vi "TemperatureSetup (SubVI).vi"() -> (0 "error out":errorcluster, 3 "Refnum out":refnum<k21>)   [LabVIEW 2016]
uses:
  <vilib>/DAQmx/create/channels.llb/DAQmx Create Channel (AI-Temperature-Thermocouple).vi
  <resource>/objmgr/daqmx.rc
  <vilib>/DAQmx/configure/timing.llb/DAQmx Timing (Sample Clock).vi
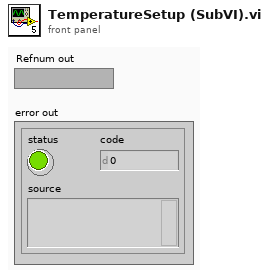
[diagram p1: front panel]
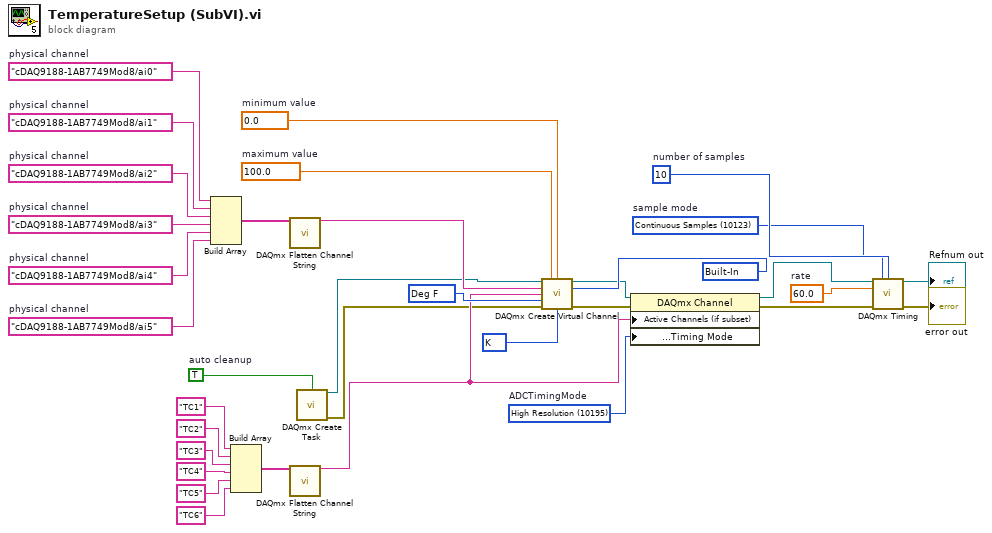
[diagram p0: block diagram]
diagram:
  w29 = "cDAQ9188-1AB7749Mod8/ai5"  # physical channel
  w28 = "cDAQ9188-1AB7749Mod8/ai4"  # physical channel
  w27 = "cDAQ9188-1AB7749Mod8/ai3"  # physical channel
  w26 = "cDAQ9188-1AB7749Mod8/ai2"  # physical channel
  w22 = "cDAQ9188-1AB7749Mod8/ai1"  # physical channel
  w21 = "cDAQ9188-1AB7749Mod8/ai0"  # physical channel
  w20 = 10144 items=["Deg C"=10143, "Deg F"=10144, "Kelvins"=10325, "Deg R"=10145, "From Custom Scale"=10065] ("units")
  w19 = 10073 items=["J"=10072, "K"=10073, "N"=10077, "R"=10082, "S"=10085, "T"=10086, "B"=10047, "E"=10055] ("thermocouple type")
  w18 = 10200 items=["Built-In"=10200, "Constant Value"=10116, "Channel"=10113] ("cjc source")
  w1 = 10123 items=["Finite Samples"=10178, "Continuous Samples"=10123, "Hardware Timed Single Point"=12522]  # sample mode
  w2 = 10  # number of samples
  w3 = 60.0  # rate
  w6 = 10195 items=["High Resolution"=10195, "High Speed"=14712, "Best 50 Hz Rejection"=14713, "Best 60 Hz Rejection"=14714]  # ADCTimingMode
  w9 = 0.0  # minimum value
  w10 = 100.0  # maximum value
  w12 = TRUE  # auto cleanup
  n1 = Build Array(w21, w22, w26, w27, w28, w29) -> (w33:string[])
  n2 = Build Array("TC1" ("name to assign"), "TC2" ("name to assign"), "TC3" ("name to assign"), "TC4" ("name to assign"), "TC5" ("name to assign"), "TC6" ("name to assign")) -> (w34:string[])
  n3 = call <vilib>:"DAQmx Flatten Channel String.vi"("names in"=w33) -> ("names out"=w16:string)  [unwired: 13 in, 1 out]
  n4 = call <vilib>:"DAQmx Flatten Channel String.vi"("names in"=w34) -> ("names out"=w17:string)  [unwired: 13 in, 1 out]
  n5 = call <vilib>:"DAQmx Create Task.vi"("auto cleanup"=w12) -> ("task out"=w11:refnum<k21>, "error out"=w13:errorcluster)  [unwired: 4 in, 9 out]
  n6 = call-poly <vilib>:"DAQmx Create Virtual Channel.vi"("task in"=w11, "maximum value"=w10, "minimum value"=w9, "physical channels"=w16, "cjc source"=w18, "name to assign"=w17, "units"=w20, "error in"=w13, "thermocouple type"=w19) -> ("task out"=w5:refnum<k21>, "error out"=w8:errorcluster)  [unwired: 5 in]
  n7 = property class="DAQmx Channel"(reference=w5, error in=w8, "Active Channels (if subset)"=w17, "Analog Input:General Properties:Digitizer/ADC:Timing Mode"=w6) -> (reference out=w4:refnum<k21>, error out=w7:errorcluster)
  n8 = call-poly <vilib>:"DAQmx Timing.vi"("task/channels in"=w4, "sample mode"=w1, "samples per channel"=w2, "rate"=w3, "error in"=w7) -> ("task out"=→"Refnum out":refnum<k21>, "error out"=→"error out":errorcluster)  [unwired: 2 in, 7 out]
